vi "SubVI_NewWindResults_001.vi"(0 "Open results in another window":bool, 1 "Results and dissimilarity":cluster{string[], "Dissimilarity":dbl[][]}, 2 "Correct?":bool[](array[boolean]), 3 "paths":path[](array[path])) -> ()   [LabVIEW 2018]
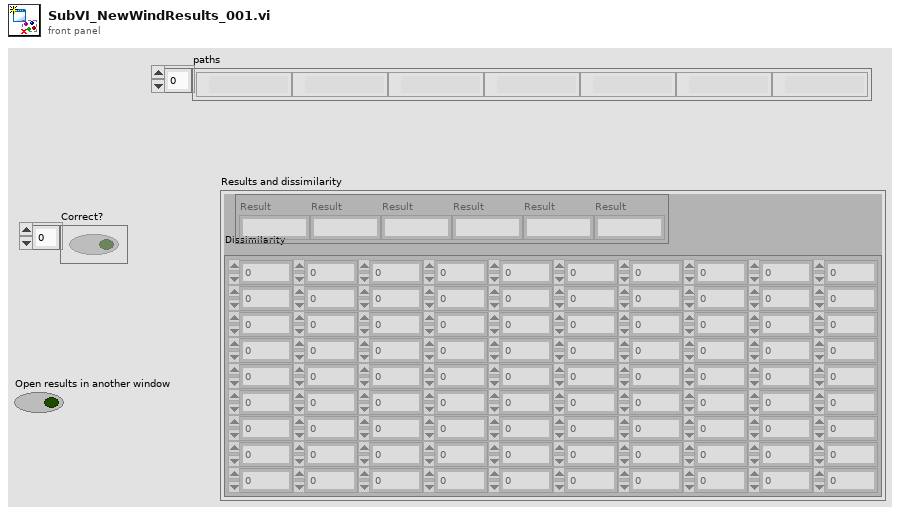
[diagram p1: front panel]
types:
  T1 = enum32{"Invalid", "Standard", "Closed", "Hidden", "Minimized", "Maximized"}
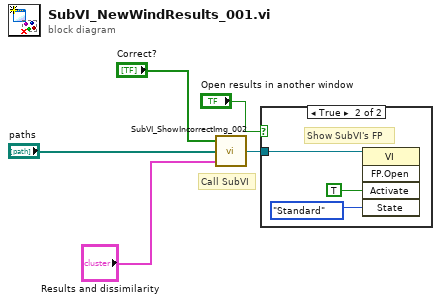
[diagram p0: block diagram]
diagram:
  # "Call SubVI"
  n1 = call "SubVI_ShowIncorrectImg_002.vi"("output cluster"="Results and dissimilarity", "selected path"="paths", "Correct?"="Correct?") -> ("This VI"=w3:refnum<vi>)
  n2 = case shown="True" "Open results in another window" {
    tunnel: w3 -> [_ w8]
    frame False {
    }
    frame True {
      # "Show SubVI's FP"
      n3 = invoke class="VI" method="FP.Open"(reference=w8, "Activate"=TRUE ("Activate?"), "State"=T1."Standard") -> ()  [unwired: 2 in, 5 out]
    }
  }
